vi "Product Mode.vi"(7 "Next Name":string, 9 "Result":bool, 10 "Mode":bool) -> (2 "Next Name Out":string)   [LabVIEW 2017]
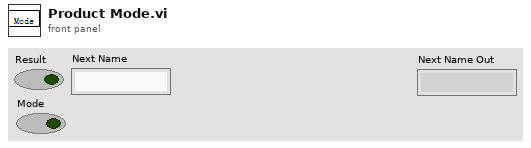
[diagram p1: front panel]
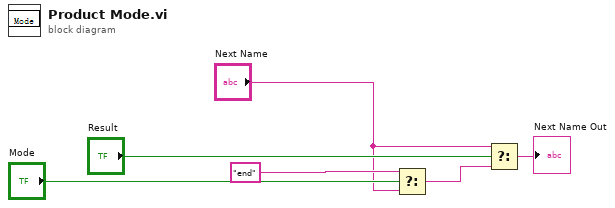
[diagram p0: block diagram]
diagram:
  n1 = Select(t="end", s="Mode", f="Next Name") -> (s? t:f=w6:string)
  n2 = Select(t="Next Name", s="Result", f=w6) -> (s? t:f=→"Next Name Out":string)
